vi "Get Target IP and Port by Node Ref.vi"(7 "Target Node In":refnum<k24>, 8 "error in (no error)":errorcluster, 11 "Custom Device Node in":refnum<k24>) -> (0 "error out":errorcluster, 1 "IP":string, 4 "Port":u16)   [LabVIEW 2011]
uses:
  NationalInstruments.VeriStand.SystemStorage
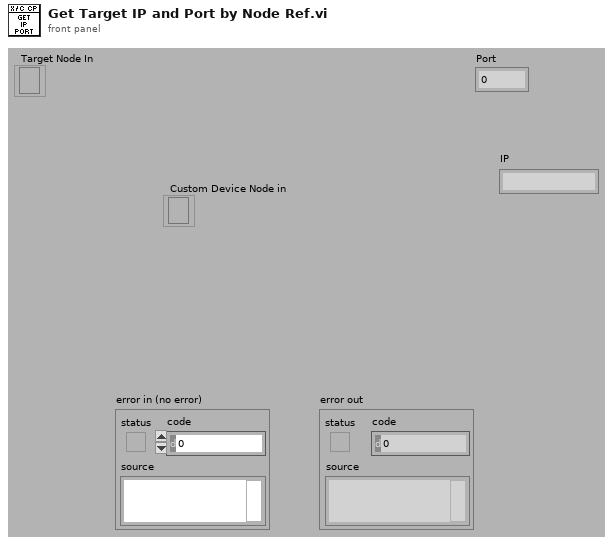
[diagram p1: front panel]
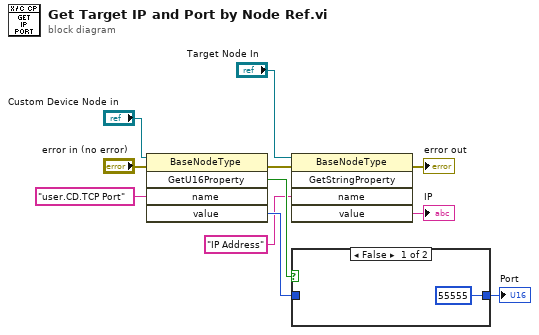
[diagram p0: block diagram]
diagram:
  n1 = invoke class="BaseNodeType" method="GetU16Property"(reference="Custom Device Node in", error in="error in (no error)", "name"="user.CD.TCP Port") -> (error out=w5:errorcluster, "GetU16Property"=w9:bool, "value"=w10:u16)  [unwired: 2 in, 2 out]
  n2 = invoke class="BaseNodeType" method="GetStringProperty"(reference="Target Node In", error in=w5, "name"="IP Address") -> (error out=→"error out":errorcluster, "value"=→"IP":string)  [unwired: 2 in, 3 out]
  n3 = case shown="False" w9 {
    tunnel: [u16 55555 ("value") w13] -> w1
    tunnel: w10 -> [_ w13]
    frame False {
    }
    frame True {
    }
  }
  "Port" <- w1
